vi "Simple CSV.vi"(0 "Filepath In":path, 2 "Mode":enum16{"Read", "Write"}(ring), 7 "Data In":string[][](array[string]), 9 "Append(T)":bool=TRUE, 11 "Error In":errorcluster) -> (4 "Filepath Out":path, 8 "Data Out":string[][](array[string]), 15 "Error Out":errorcluster)   [LabVIEW 2019]
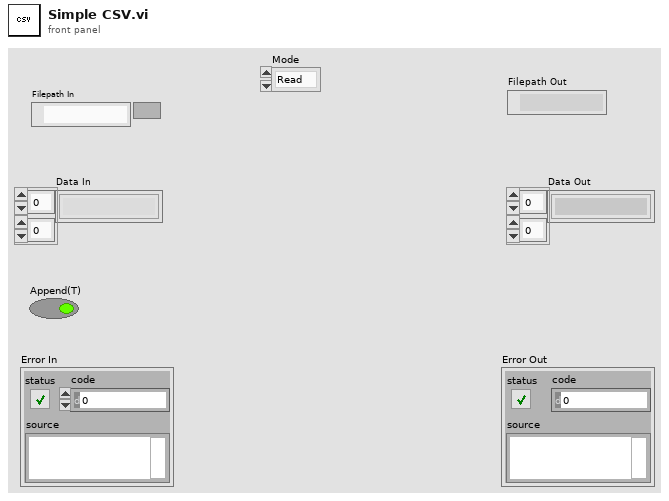
[diagram p1: front panel]
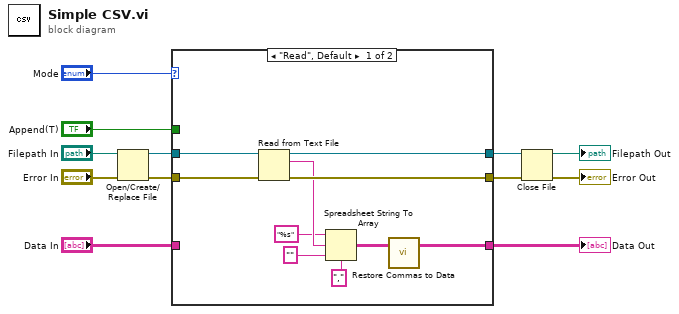
[diagram p0: block diagram]
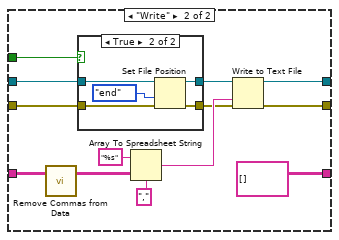
[diagram p2: hidden frame]
diagram:
  n1 = Open/Create/Replace File(file path (use dialog)="Filepath In", error in="Error In") -> (refnum out=w11:refnum<file>, error out=w10:errorcluster)  [unwired: 4 in, 1 out]
  n2 = case shown="\"Read\", Default" "Mode" {
    tunnel: w11 -> [w22 w29]
    tunnel: w10 -> [w21 w27]
    tunnel: [w20 w35] -> w9
    tunnel: [w19 w34] -> w8
    tunnel: [w13 string[][] []] -> w7
    tunnel: "Data In" -> [_ w24]
    tunnel: "Append(T)" -> [_ w30]
    frame "Read", Default {
      n3 = Read from Text File(file (use dialog)=w22, error in=w21) -> (refnum out=w20:refnum<file>, text=w18:string, error out=w19:errorcluster)  [unwired: 2 in, 1 out]
      n4 = Spreadsheet String To Array(delimiter (Tab)=",", format string="%s", spreadsheet string=w18, array type (2D Dbl)="") -> (array=w14:string[][])
      n5 = call "Restore Commas to Data.vi"("Data In"=w14) -> ("Data Out"=w13:string[][])  [unwired: 5 in]
    }
    frame "Write" {
      n6 = call "Remove Commas from Data.vi"("Data In"=w24) -> ("Data Out"=w23:string[][])  [unwired: 5 in]
      n7 = case shown="True" w30 {
        tunnel: w29 -> [w37 w42]
        tunnel: [w37 w41] -> w28
        tunnel: w27 -> [w36 w40]
        tunnel: [w36 w39] -> w26
        frame False {
        }
        frame True {
          n8 = Set File Position(refnum=w42, from (0:start)=enum16{"start", "end", "current"}."end", error in=w40) -> (refnum out=w41:refnum<file>, error out=w39:errorcluster)  [unwired: 1 in]
        }
      }
      n9 = Array To Spreadsheet String(delimiter (Tab)=",", array=w23, 3:"%s" ("format string")) -> (spreadsheet string=w32:string)
      n10 = Write to Text File(file (use dialog)=w28, text=w32, error in=w26) -> (refnum out=w35:refnum<file>, error out=w34:errorcluster)  [unwired: 1 in, 1 out]
    }
  }
  "Data Out" <- w7
  n11 = Close File(refnum=w9, error in=w8) -> (path=→"Filepath Out":path, error out=→"Error Out":errorcluster)
